vi "Measurement Logic.vi"() -> ()   [LabVIEW 2020, in "Keysight 34401A DMM Measurement.lvlib"]
uses:
  Keysight 34401A DMM Measurement.lvlib
  Keysight 34401A DMM Instrument/Keysight 34401A DMM Instrument.lvlib
  Keysight 34401A DMM Instrument/Initialize Sessions - 1Sess.vi
  <vilib>/Plug-In SDKs/Clients/Session Management V1/Session Reservation/Session Reservation.lvclass
  <vilib>/Plug-In SDKs/Measurements/Measure Call Context/Measure Call Context.lvclass
  Measurement Configuration.ctl
  Measurement Results.ctl
  subVIs/Keysight 34401A Function.ctl
panel:
  out "measure call context out":refnum<class "Measure Call Context.lvclass">
  in  "measure call context in":refnum<class "Measure Call Context.lvclass">
  out "measurement results":T1
  in  "measurement configuration":T2
  out "error out":errorcluster
  in  "error in":errorcluster
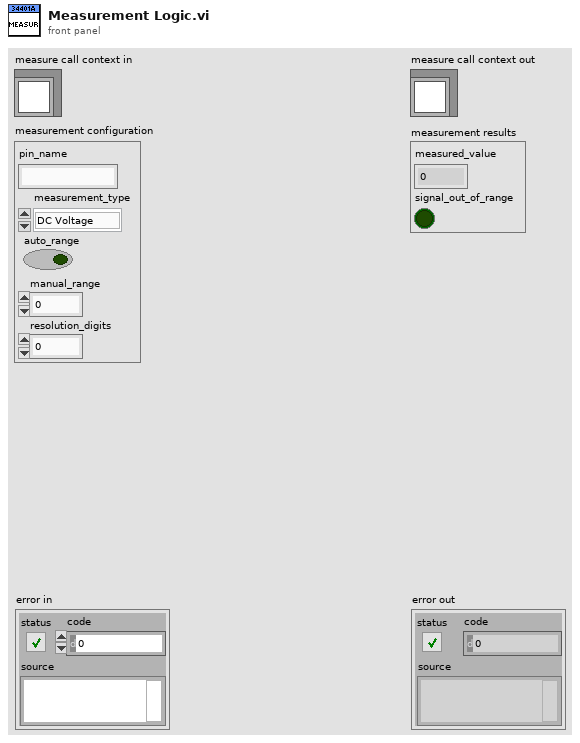
[diagram p1: front panel]
types:
  T1 = typedef "Keysight 34401A DMM Measurement.lvlib/Measurement Results.ctl" = cluster{"measured_value":dbl, "signal_out_of_range":bool}
  T2 = typedef "Keysight 34401A DMM Measurement.lvlib/Measurement Configuration.ctl" = cluster{"pin_name":string, "measurement_type":T3, "auto_range":bool, "manual_range":dbl, "resolution_digits":dbl}
  T3 = typedef "Keysight 34401A DMM Measurement.lvlib/Keysight 34401A Function.ctl" = enum32{"DC Voltage", "AC Voltage", "2 - Wire Resistance", "4 - Wire Resistance", "DC Current", "AC Current", "Frequency", "Period", "Continuity", "Diode Checking", "VDC:VDC Ratio", "Temperature", "Capacitance"}
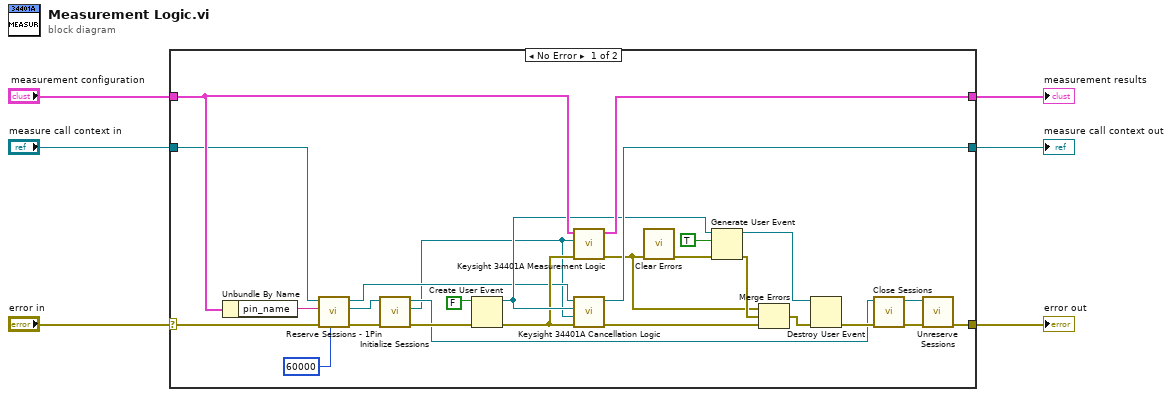
[diagram p0: block diagram]
diagram:
  n1 = case shown="No Error" "error in" {
    selector: "error in" -> [w19 w35]
    tunnel: "measure call context in" -> [w20 w34]
    tunnel: [w15 w35] -> w5
    tunnel: "measurement configuration" -> [w32 _]
    tunnel: [w33 _] -> w3
    tunnel: [w31 w34] -> w2
    frame No Error {
      n2 = Unbundle By Name(w32) -> ("pin_name"=w18:string)
      n3 = call <vilib>:"Reserve Sessions - 1Pin.vi"("timeout (ms)"=60000 ("timeout in milliseconds"), "error in"=w19, "pin or relay name"=w18, "measurement context in"=w20) -> ("error out"=w11:errorcluster, "session reservation out"=w9:refnum<class "Session Reservation.lvclass">, "measurement context out"=w16:refnum<class "Measure Call Context.lvclass">)  [unwired: 5 in]
      n4 = call-poly "Initialize Sessions.vi"("error in"=w11, "session reservation in"=w9) -> ("error out"=w10:errorcluster, "session"=w7:refnum<visa-resource-name>, "session reservation out"=w8:refnum<class "Session Reservation.lvclass">)  [unwired: 6 in, 1 out]
      n5 = Create User Event(user event datatype=FALSE ("measurement complete"), error in=w10) -> (user event=w27:refnum<user-event>, error out=w25:errorcluster)
      n6 = call "Keysight 34401A Measurement Logic.vi"("error in (no error)"=w25, "session"=w7, "measurement configuration"=w32) -> ("error out"=w21:errorcluster, "measurement results"=w33:T1)  [unwired: 7 in]
      n7 = call "Keysight 34401A Cancellation Logic.vi"("error in (no error)"=w25, "session"=w7, "measurement complete"=w27, "MeasurementContext in"=w16) -> ("error out"=w30:errorcluster, "MeasurementContext out"=w31:refnum<class "Measure Call Context.lvclass">)  [unwired: 6 in]
      n8 = call <vilib>:"Clear Errors.vi"("error in (no error)"=w21) -> ("error out"=w22:errorcluster)  [unwired: 5 in, 1 out]
      n9 = Generate User Event(user event=w27, event data cluster=TRUE ("event data"), error in=w22) -> (user event out=w23:refnum<user-event>, error out=w26:errorcluster)  [unwired: 1 in]
      n10 = Merge Errors(w21, w26, w30) -> (w24:errorcluster)
      n11 = Destroy User Event(user event=w23, error in=w24) -> (error out=w14:errorcluster)
      n12 = call <vilib>:"Close Sessions.vi"("error in"=w14, "session reservation in"=w8) -> ("error out"=w13:errorcluster, "session reservation out"=w12:refnum<class "Session Reservation.lvclass">)  [unwired: 8 in]
      n13 = call <vilib>:"Unreserve Sessions.vi"("error in"=w13, "session reservation in"=w12) -> ("error out"=w15:errorcluster)  [unwired: 9 in]
    }
    frame Error {
    }
  }
  "error out" <- w5
  "measurement results" <- w3
  "measure call context out" <- w2
